vi "Memory.Pointer.Allocate (32-bit).vi"(8 "error in (no error)":errorcluster, 11 "size":i32 format="%d bytes") -> (0 "error out":errorcluster, 3 "Pointer out":refnum<class "Memory.Pointer.lvclass">)   [LabVIEW 2016, in "LabVIEW Memory Manager.lvlib" / "Memory.Pointer.lvclass"]
uses:
  Memory.Pointer.lvclass
  Memory.Pointer.lvclass/Memory.Pointer.ctl
  Accessors/Memory.Pointer.Set Address.vi
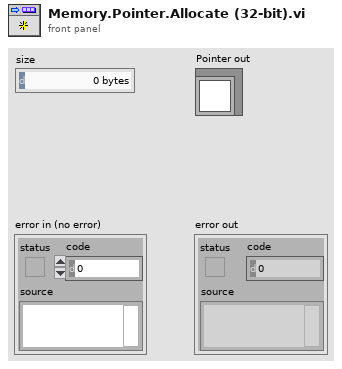
[diagram p1: front panel]
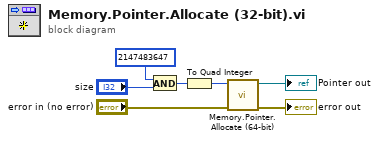
[diagram p0: block diagram]
diagram:
  n1 = And(x=2147483647 ("y"), y="size") -> (x .and. y?=w1:i32)
  n2 = To Quad Integer(1:w1) -> (0:w4:i64)
  n3 = call "Memory.Pointer.Allocate (64-bit).vi"("error in (no error)"="error in (no error)", "size"=w4) -> ("error out"=→"error out":errorcluster, "Pointer out"=→"Pointer out":refnum<class "Memory.Pointer.lvclass">)  [unwired: 8 in]
